vi "ParseURI.vi"(8 "error in":errorcluster, 11 "URI":string="https://tools.ietf.org:80/html/rfc3986?query=test&query2=test2#appendix-A") -> (0 "error out":errorcluster, 1 "path":string, 2 "authority":string, 3 "scheme":string, 4 "query":string, 6 "fragment":string)   [LabVIEW 2013, in "URI.lvlib"]
uses:
  <vilib>/regexp/Match Regular Expression.xnode
  URI.lvlib
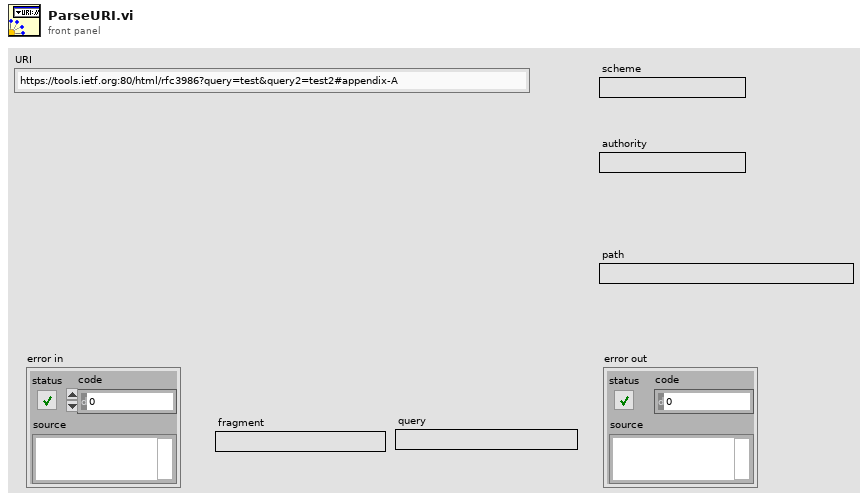
[diagram p1: front panel]
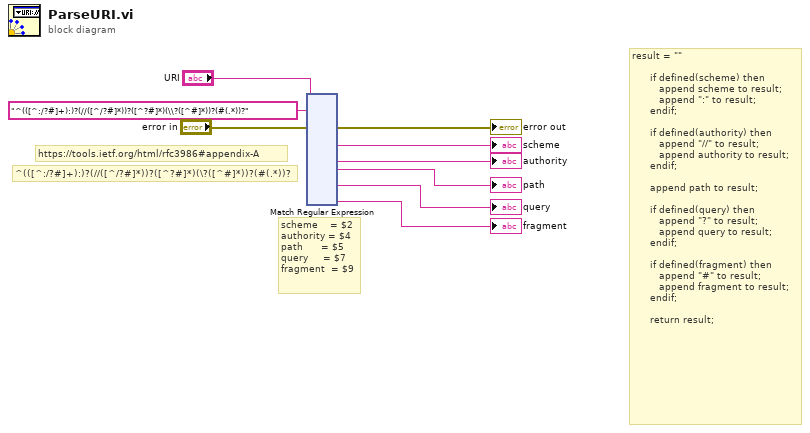
[diagram p0: block diagram]
diagram:
  # "https://tools.ietf.org/html/rfc3986#appendix-A"
  # "result = \"\"\n\n      if defined(scheme) then\n         append scheme to result;\n         append \":\" to result;\n      endif;\n\n      if defined(authority) then\n         append \"//\" to result;\n         append authority to result;\n      endif;\n\n      append path to result;\n\n      if defined(query) then\n         append \"?\" to result;\n         append query to result;\n      endif;\n\n      if defined(fragment) then\n         append \"#\" to result;\n         append fragment to result;\n      endif;\n\n      return result;"
  # "scheme    = $2\nauthority = $4\npath      = $5\nquery     = $7\nfragment  = $9"
  # "^(([^:/?#]+):)?(//([^/?#]*))?([^?#]*)(\\?([^#]*))?(#(.*))?"
  n1 = xnode "Match Regular Expression"("input string"="URI", "regular expression"="^(([^:/?#]+):)?(//([^/?#]*))?([^?#]*)(\\?([^#]*))?(#(.*))?", "error in"="error in") -> ("error out"=→"error out":errorcluster, "submatch 2"=→"scheme":string, "submatch 4"=→"authority":string, "submatch 5"=→"path":string, "submatch 7"=→"query":string, "submatch 9"=→"fragment":string)  [unwired: 3 in, 8 out]
